vi "Parse Thermostate Mode.vi"(8 "Error In":errorcluster, 9 "Data":string, 10 "Device ID":string, 11 "Nest Config":T2) -> (0 "Error Out":errorcluster, 1 "Data":string, 2 "Thermostat Mode":T1, 3 "Nest Config":T2)   [LabVIEW 2013, in "LMH-Nest.lvlib"]
doc: "Get the current thermostat mode (heat / cool)."
uses:
  LMH-Nest.lvlib
  Type Defs/Nest Config.ctl
  <vilib>/httpClient/ClientHandle.ctl
  Type Defs/Session Data.ctl
  Type Defs/Thermostat Mode.ctl
  <vilib>/httpClient/LabVIEWHTTPClient.lvlib
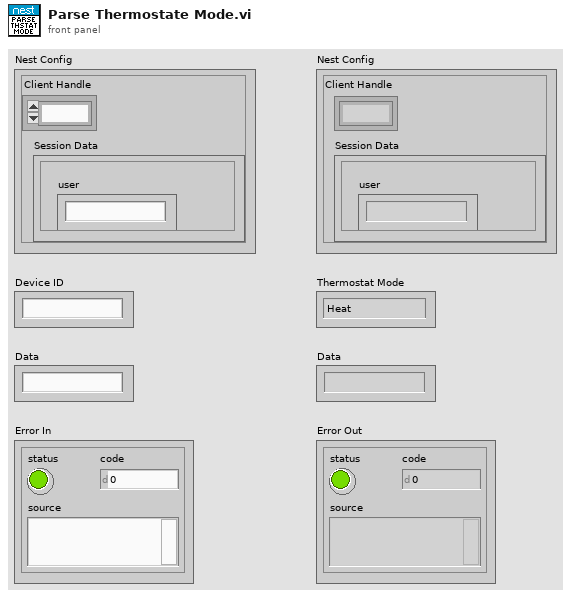
[diagram p1: front panel]
types:
  T1 = typedef "LMH-Nest.lvlib/Thermostat Mode.ctl" = enum16{"Heat", "Cool", "Heat / Cool"}
  T2 = typedef "LMH-Nest.lvlib/Nest Config.ctl" = cluster{"Client Handle":T3, "Session Data":T4}
  T3 = typedef "LabVIEWHTTPClient.lvlib/ClientHandle.ctl" = refnum<k1>
  T4 = typedef "LMH-Nest.lvlib/Session Data.ctl" = cluster{"is_superuser":bool, "is_staff":bool, "urls":cluster{"transport_url":string, "rubyapi_url":string, "weather_url":string, "log_upload_url":string, "support_url":string}, "limits":cluster{"thermostats_per_structure":u32, "structures":u32, "thermostats":u32, "smoke_detectors":u32, "smoke_detectors_per_structure":u32}, "access_token":string, "userid":string, "expires_in":string, "email":string, "user":string, "language":string}
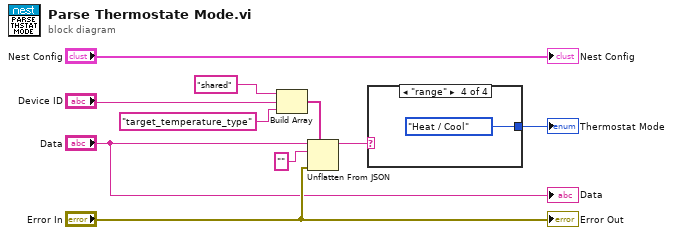
[diagram p0: block diagram]
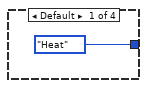
[diagram p2: hidden frame]
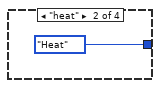
[diagram p3: hidden frame]
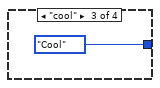
[diagram p4: hidden frame]
diagram:
  n1 = Build Array("shared", "Device ID", "target_temperature_type" ("element")) -> (w8:string[])
  n2 = Unflatten From JSON(path=w8, JSON string="Data", type and defaults="" ("element"), error in (no error)="Error In") -> (value=w2:string)  [unwired: 3 in, 1 out]
  n3 = case shown="\"range\"" w2 {
    tunnel: [Thermostat_Mode."Heat" ("Thermostat Mode") Thermostat_Mode."Heat" ("Thermostat Mode") Thermostat_Mode."Cool" ("Thermostat Mode") Thermostat_Mode."Heat / Cool" ("Thermostat Mode")] -> w1
    frame Default {
    }
    frame "heat" {
    }
    frame "cool" {
    }
    frame "range" {
    }
  }
  "Thermostat Mode" <- w1
  "Nest Config" <- "Nest Config"
  "Error Out" <- "Error In"
  "Data" <- "Data"
